vi "teste-math.vi"() -> ()   [LabVIEW 2014]
uses:
  <vilib>/Analysis/NI_AALBase.lvlib
panel:
  out "Waveform Graph":dbl[](graph)
  out "variance":dbl format="%0.5f"
  out "standard deviation":dbl format="%0.5f"
  out "mean":dbl format="%0.5f"
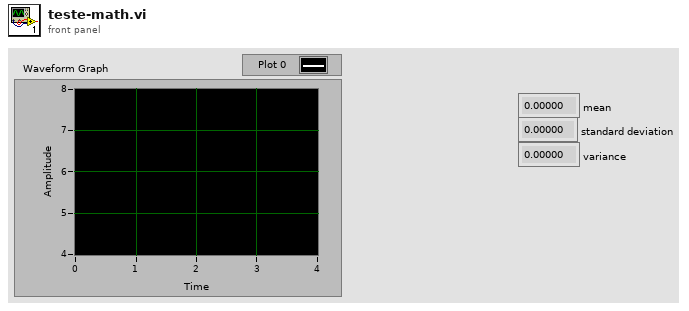
[diagram p1: front panel]
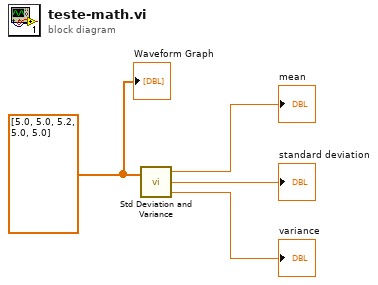
[diagram p0: block diagram]
diagram:
  w1 = dbl[] [5.0, 5.0, 5.2, 5.0, 5.0]
  n1 = call <vilib>:"Std Deviation and Variance.vi"("X"=w1) -> ("mean"=→"mean":dbl, "standard deviation"=→"standard deviation":dbl, "variance"=→"variance":dbl)  [unwired: 1 in]
  "Waveform Graph" <- w1
